vi "数据写入database.vi"(9 "data":variant, 10 "columns":string[](array[string]), 11 "table":string) -> (1 "error out":errorcluster)   [LabVIEW 2016, in "斯坦道CODMn.lvlib"]
uses:
  <vilib>/Utility/sysdir.llb/System Directory Type.ctl
  <vilib>/addons/database/Connection.llb/DB Tools Open Connec (String).vi
  <vilib>/addons/database/Connection.llb/Conn Execute.vi
  <vilib>/addons/database/Recordset.llb/Rec Destroy - Connection.vi
  <vilib>/addons/database/Recordset.llb/Rec Fetch Recordset Data (R).vi
  <vilib>/addons/database/NI_Database_API.lvlib
panel:
  out "为空？":bool
  in  "error in (no error)":errorcluster
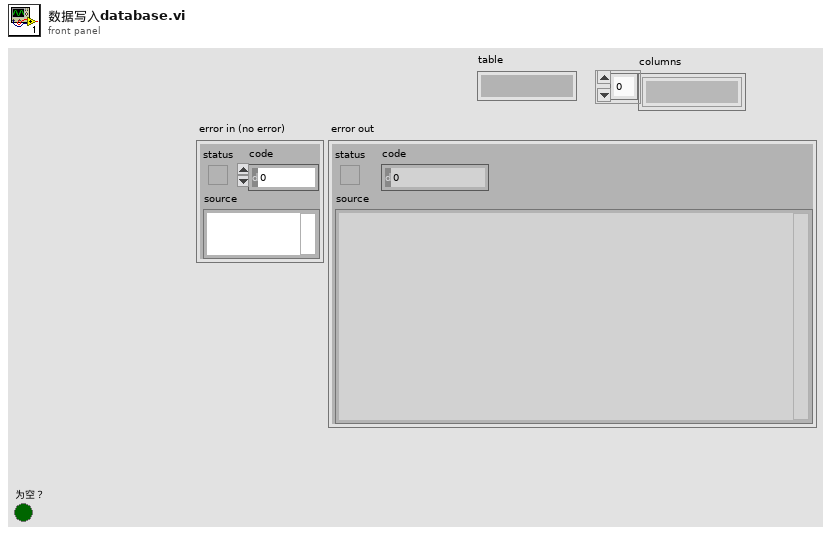
[diagram p1: front panel]
types:
  T1 = cluster{"时间":timestamp, "测量模式":string, "数据类型":string, "检测值":sgl, "单位":string, "数据标识":string, "因子编码":string, "标样参考值":sgl, "ORP-A":sgl, "ORP-B":sgl, "ORP-K":sgl, "COD滴定值":sgl, "高锰酸钾滴定数":sgl, "温度":sgl, "量程":sgl}
  T2 = typedef "System Directory Type.ctl" = i32
  T3 = typedef "NI_Database_API.lvlib/Conn ObjectReference.ctl" = refnum<k1>
  T4 = typedef "NI_Database_API.lvlib/Rec ObjectReference.ctl" = refnum<k1>
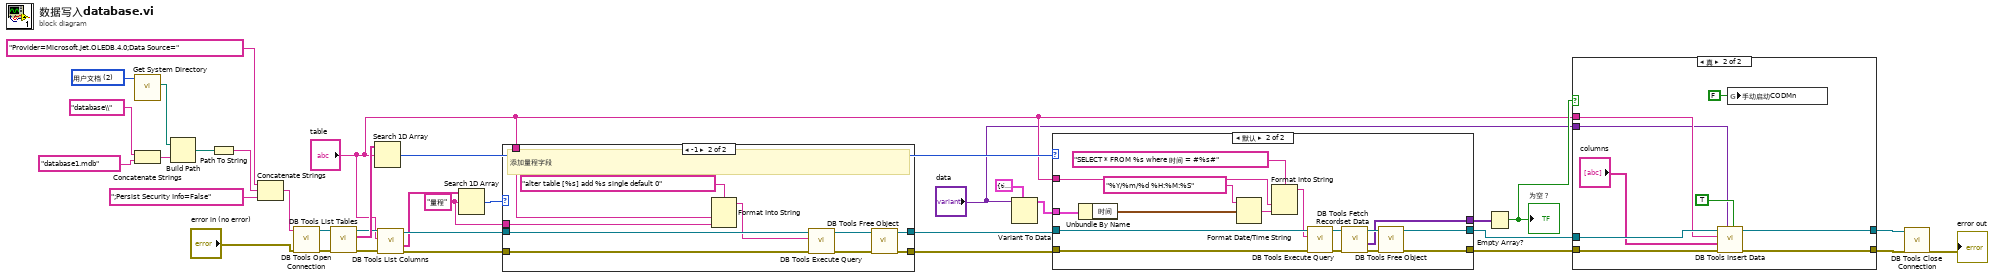
[diagram p0: block diagram]
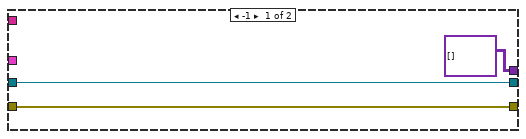
[diagram p4: hidden frame]
diagram:
  w7 = "量程" ("元素")
  w35 = T2 2 items=["用户目录"=0, "用户桌面"=1, "用户文档"=2, "用户应用程序数据"=3, "用户设置"=4, "用户临时目录"=5, "公共文档"=6, "公共应用程序数据"=7, "公共设置"=8, "公共缓存"=13, "系统核心库"=9, "系统安装库"=10, "应用程序文件"=11, "启动盘根目录"=12] ("system directory type")
  n1 = call <vilib>:"Get System Directory.vi"("system directory type"=w35) -> ("system directory"=w33:path)  [unwired: 10 in]
  n2 = Concatenate Strings("database\\" ("condition"), "database1.mdb" ("字符串")) -> (w27:string)
  n3 = Build Path(base path=w33, name or relative path=w27) -> (appended path=w32:path)
  n4 = Path To String(path=w32) -> (string=w31:string)
  n5 = Concatenate Strings("Provider=Microsoft.Jet.OLEDB.4.0;Data Source=" ("condition"), w31, ";Persist Security Info=False" ("condition")) -> (w29:string)
  n6 = call-poly <vilib>:"DB Tools Open Connection.vi"("error in (no error)"="error in (no error)", "connection information"=w29) -> ("error out"=w24:errorcluster, "connection reference"=w25:T3)  [unwired: 6 in]
  n7 = call <vilib>:"DB Tools List Tables.vi"("error in (no error)"=w24, "connection reference"=w25) -> ("error out"=w12:errorcluster, "tables"=w23:string[], "connection reference out"=w13:T3)  [unwired: 3 in]
  n8 = Search 1D Array(1D array=w23, element="table") -> (index of element=w22:i32)  [unwired: 1 in]
  n9 = call <vilib>:"DB Tools List Columns.vi"("error in (no error)"=w12, "table"="table", "connection reference"=w13) -> ("error out"=w10:errorcluster, "columns"=w9:string[], "connection reference out"=w11:T3)  [unwired: 1 in, 1 out]
  n10 = Search 1D Array(1D array=w9, element=w7) -> (index of element=w8:i32)  [unwired: 1 in]
  n11 = case shown="-1" w8 {
    tunnel: w11 -> [w37 w45]
    tunnel: w10 -> [w36 w44]
    tunnel: "table" -> [_ w42]
    tunnel: w7 -> [_ w41]
    tunnel: [w37 w39] -> w6
    tunnel: [w36 w38] -> w5
    frame 0, Default {
    }
    frame -1 {
      # "添加量程字段"
      n12 = Format Into String(format string="alter table [%s] add %s single default 0", w42, w41) -> (resulting string=w40:string)  [unwired: 2 in, 1 out]
      n13 = call-poly <vilib>:"DB Tools Execute Query.vi"("error in (no error)"=w44, "SQL query"=w40, "connection reference"=w45) -> ("error out"=w46:errorcluster, "recordset reference"=w47:T4)  [unwired: 5 in]
      n14 = call-poly <vilib>:"DB Tools Free Object.vi"("error in (no error)"=w46, "recordset reference"=w47) -> ("error out"=w38:errorcluster, "connection reference"=w39:T3)  [unwired: 8 in]
    }
  }
  n15 = Variant To Data(type=T1 {"时间"=timestamp(0 s since 1904-01-01), "测量模式"="", "数据类型"="", "检测值"=0.0, "单位"="", "数据标识"="", "因子编码"="", "标样参考值"=0.0, "ORP-A"=0.0, "ORP-B"=0.0, "ORP-K"=0.0, "COD滴定值"=0.0, "高锰酸钾滴定数"=0.0, "温度"=0.0, "量程"=0.0} ("data"), Variant="data") -> (data=w1:T1)  [unwired: 1 in, 1 out]
  n16 = case shown="默认" w22 {
    tunnel: [variant[][] [] ("recordset data") w62] -> w26
    tunnel: [w50 w61] -> w19
    tunnel: [w49 w60] -> w20
    tunnel: w6 -> [w50 w59]
    tunnel: w5 -> [w49 w58]
    tunnel: "table" -> [_ w57]
    tunnel: w1 -> [_ w52]
    frame -1 {
    }
    frame Default {
      n17 = Unbundle By Name(w52) -> ("时间"=w55:timestamp)
      n18 = Format Date/Time String(time format string (%c)="%Y/%m/%d %H:%M:%S" ("时间格式字符串(%c)"), seconds (now)=w55) -> (date/time string=w53:string)  [unwired: 1 in]
      n19 = Format Into String(format string="SELECT * FROM %s where 时间 = #%s#" ("格式字符串"), w57, w53) -> (resulting string=w56:string)  [unwired: 2 in, 1 out]
      n20 = call-poly <vilib>:"DB Tools Execute Query.vi"("error in (no error)"=w58, "SQL query"=w56, "connection reference"=w59) -> ("error out"=w63:errorcluster, "recordset reference"=w66:T4)  [unwired: 5 in]
      n21 = call-poly <vilib>:"DB Tools Fetch Recordset Data.vi"("error in (no error)"=w63, "recordset reference"=w66) -> ("error out"=w64:errorcluster, "recordset data"=w62:variant[][], "recordset reference out"=w65:T4)  [unwired: 3 in]
      n22 = call-poly <vilib>:"DB Tools Free Object.vi"("error in (no error)"=w64, "recordset reference"=w65) -> ("error out"=w60:errorcluster, "connection reference"=w61:T3)  [unwired: 8 in]
    }
  }
  n23 = Empty Array?(array=w26) -> (empty?=w21:bool)
  "为空？" <- w21
  n24 = case shown="真" w21 {
    tunnel: "table" -> [_ w72]
    tunnel: "data" -> [_ w71]
    tunnel: w20 -> [w67 w77]
    tunnel: w19 -> [w68 w76]
    tunnel: [w68 w74] -> w18
    tunnel: [w67 w73] -> w17
    frame False {
    }
    frame True {
      n25 = call <vilib>:"DB Tools Insert Data.vi"("create table? (F)"=TRUE, "data"=w71, "error in (no error)"=w77, "columns"="columns", "table"=w72, "connection reference"=w76) -> ("error out"=w73:errorcluster, "connection reference out"=w74:T3)  [unwired: 4 in]
      n26 = global write "CODMN外部API.vi" "手动启动CODMn"(FALSE ("手动启动CODMn")) -> ()
    }
  }
  n27 = call <vilib>:"DB Tools Close Connection.vi"("error in (no error)"=w17, "connection reference"=w18) -> ("error out"=→"error out":errorcluster)  [unwired: 5 in]
